vi "CC Data Logging Loop.vi"(11 "user event":refnum<user-event>) -> ()   [LabVIEW 2024]
uses:
  hk-channel-class/hk-channel-class/HK Table/HK Table.lvclass
  Subsystems/SS cluster Data Queue type.ctl
  CC enum Current Values Action.ctl
  Subsystems/SS cluster New Image Data.ctl
  typedefs/CC cluster Alarm Data.ctl
  typedefs/CC enum Alarm Action.ctl
  typedefs/CC cluster System Settings.ctl
  hk-channel-class/hk-channel-class/HK Item/HK Item.lvclass
panel:
  out "error out":errorcluster
  in  "error in (no error)":errorcluster
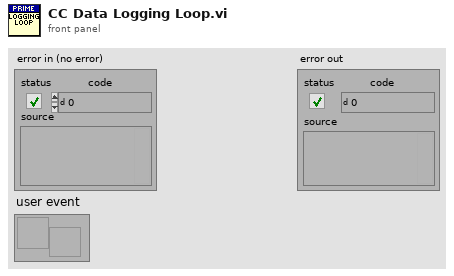
[diagram p1: front panel]
types:
  T1 = cluster{"HK Channels":refnum<class "HK Table.lvclass">, "Data Q":refnum<queue>, "user event":refnum<user-event>}
  T2 = typedef "CC enum Current Values Action.ctl" = enum16{"Init", "Write Item", "Write Array", "Read Item", "Read Array", "Read All", "Add Channels", "New File", "Add Message", "Get Current Values", "Close"}
  T3 = typedef "SS cluster New Image Data.ctl" = cluster{"Frame number":i32, "Detector #":u16, "FITS file":path, "File size":i64, "Image Type":string}
  T4 = typedef "CC enum Alarm Action.ctl" = enum16{"Init", "Add Alarm", "Get Alarms", "Clear Alarm", "Clear All Alarms"}
  T5 = typedef "CC cluster Alarm Data.ctl" = cluster{"Measured Value":dbl, "Alarm Low":dbl, "Alarm High":dbl, "Message":string, "Source":string}
  T6 = typedef "SS cluster Data Queue type.ctl" = cluster{"Source":string, "Type":string, "Data":variant}
  T7 = typedef "CC cluster System Settings.ctl" = cluster{"HK Table Name":string, "Images Folder":path, "Obs File":path}
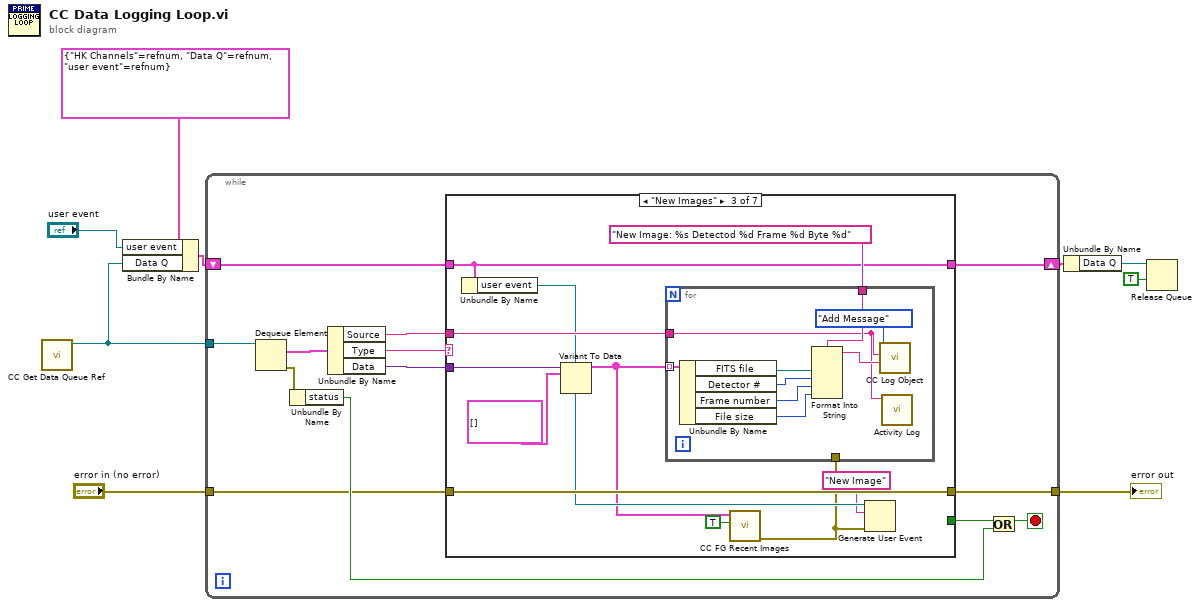
[diagram p0: block diagram]
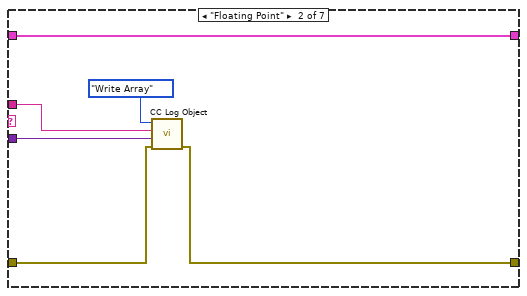
[diagram p3: hidden frame]
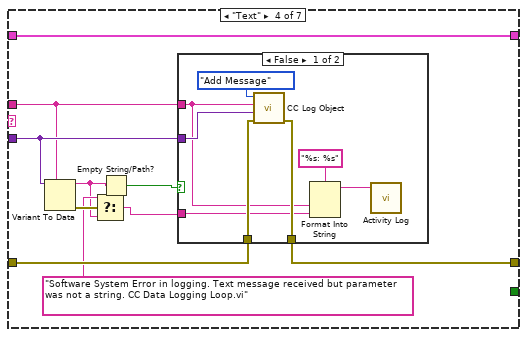
[diagram p4: hidden frame]
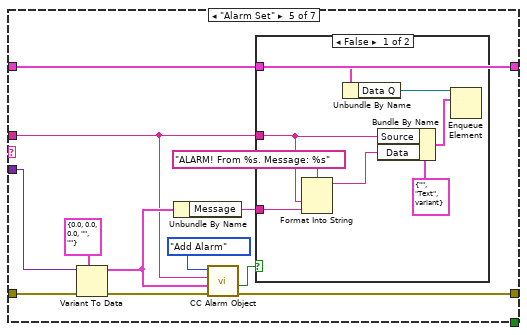
[diagram p6: hidden frame]
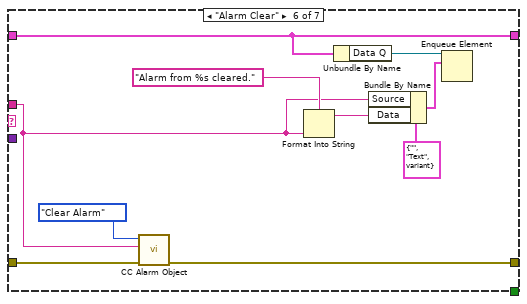
[diagram p8: hidden frame]
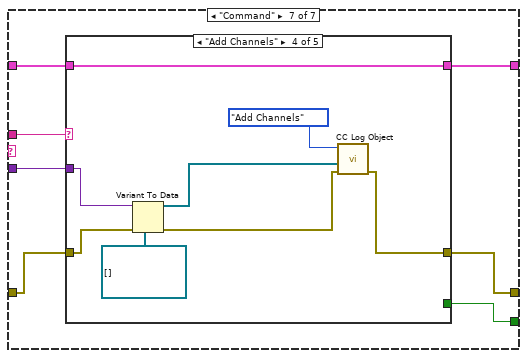
[diagram p9: hidden frame]
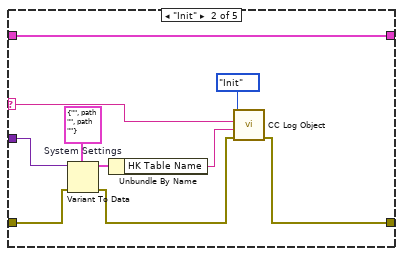
[diagram p11: hidden frame]
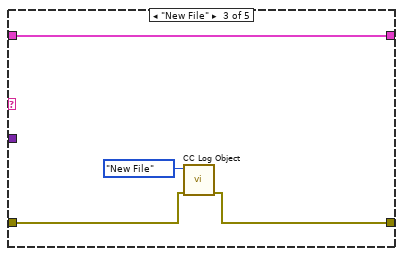
[diagram p12: hidden frame]
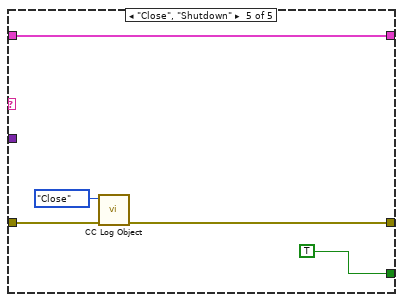
[diagram p13: hidden frame]
diagram:
  n1 = call "CC Get Data Queue Ref.vi"() -> ("Data Q"=w7:refnum<queue>)  [unwired: 10 in, 1 out]
  n2 = Bundle By Name(cluster=T1 {"HK Channels"=refnum, "Data Q"=refnum, "user event"=refnum}, "user event"="user event", "Data Q"=w7) -> (w5:T1)
  n3 = while {
    tunnel: w7 -> [w22]
    shift-right: [w12] -> w4
    shift-left: w5 -> [w16]
    tunnel: "error in (no error)" -> [w17]
    tunnel: [w11] -> w8
    stop <- w20 stop-if-true
    n4 = Dequeue Element(queue=w22) -> (element=w21:T6, error out=w19:errorcluster)  [unwired: 2 in, 2 out]
    n5 = Unbundle By Name(w19) -> ("status"=w18:bool)
    n6 = Unbundle By Name(w21) -> ("Source"=w14:string, "Type"=w15:string, "Data"=w13:variant)
    n7 = case shown="\"New Images\"" w15 {
      tunnel: w13 -> [_ w28 w41 w57 w80 _ w102]
      tunnel: w16 -> [w24 w27 w36 w60 w74 w90 w105]
      tunnel: [w24 w27 w36 w60 w74 w90 w104] -> w12
      tunnel: w14 -> [_ w29 w38 w56 w72 w89 w99]
      tunnel: w17 -> [w23 w26 w37 w59 w77 w96 w103]
      tunnel: [w23 w25 w37 w58 w75 w97 w101] -> w11
      tunnel: [_ _ _ _ _ _ w100] -> w10
      frame "False", Default {
      }
      frame "Floating Point" {
        n8 = call "CC Log Object.vi"("error in (no error)"=w26, "Data"=w28, "Source"=w29, "Action"=CC_enum_Current_Values_Action."Write Array") -> ("error out"=w25:errorcluster)  [unwired: 5 in, 2 out]
      }
      frame "New Images" {
        n9 = Unbundle By Name(w36) -> ("user event"=w35:refnum<user-event>)
        n10 = Variant To Data(type=T3[] [], Variant=w41) -> (data=w33:T3[])  [unwired: 1 in, 1 out]
        n11 = call "CC FG Recent Images.vi"("Write"=TRUE, "Recent Images"=w33) -> ("error out"=w31:errorcluster)  [unwired: 8 in, 1 out]
        n12 = for {
          tunnel: w33 -> [w50] mode=indexing
          tunnel: "New Image: %s Detectod %d Frame %d Byte %d" ("format string") -> [w49]
          tunnel: w38 -> [w42]
          tunnel: w31 -> [_]
          n13 = Unbundle By Name(w50) -> ("FITS file"=w48:path, "Detector #"=w47:u16, "Frame number"=w46:i32, "File size"=w45:i64)
          n14 = Format Into String(format string=w49, w48, w47, w46, w45) -> (resulting string=w43:string)  [unwired: 2 in, 1 out]
          n15 = call "CC Log Object.vi"("Data"=w43, "Source"=w42, "Action"=CC_enum_Current_Values_Action."Add Message") -> ()  [unwired: 6 in, 3 out]
          n16 = call "Activity Log.vi"("Message Log Entry"=w42) -> ()  [unwired: 9 in, 2 out]
        }
        n17 = Generate User Event(user event=w35, event data cluster="New Image" ("event data"), error in=w31) -> ()  [unwired: 1 in, 2 out]
      }
      frame "Text" {
        n18 = Variant To Data(type=w56, Variant=w57) -> (data=w52:string, error out=w55:errorcluster)  [unwired: 1 in]
        n19 = Select(t="Software System Error in logging. Text message received but parameter was not a string. CC Data Logging Loop.vi", s=w55, f=w52) -> (s? t:f=w54:string)
        n20 = Empty String/Path?(string/path=w52) -> (empty?=w51:bool)
        n21 = case shown="False" w51 {
          tunnel: w59 -> [w67 w69]
          tunnel: [w66 w69] -> w58
          tunnel: w57 -> [w65 _]
          tunnel: w56 -> [w63 _]
          tunnel: w54 -> [w61 _]
          frame False {
            n22 = call "CC Log Object.vi"("error in (no error)"=w67, "Data"=w65, "Source"=w63, "Action"=CC_enum_Current_Values_Action."Add Message") -> ("error out"=w66:errorcluster)  [unwired: 5 in, 2 out]
            n23 = Format Into String(format string="%s: %s", w63, w61) -> (resulting string=w62:string)  [unwired: 2 in, 1 out]
            n24 = call "Activity Log.vi"("Message Log Entry"=w62) -> ()  [unwired: 9 in, 2 out]
          }
          frame True {
          }
        }
      }
      frame "Alarm Set" {
        n25 = Variant To Data(error in=w77, type=T5 {"Measured Value"=0.0, "Alarm Low"=0.0, "Alarm High"=0.0, "Message"="", "Source"=""}, Variant=w80) -> (data=w73:T5, error out=w76:errorcluster)
        n26 = Unbundle By Name(w73) -> ("Message"=w71:string)
        n27 = call "CC Alarm Object.vi"("error in (no error)"=w76, "Alarm"=w73, "Source"=w72, "Alarm Action"=CC_enum_Alarm_Action."Add Alarm") -> ("error out"=w75:errorcluster, "key already included?"=w70:bool)  [unwired: 4 in, 2 out]
        n28 = case shown="False" w70 {
          tunnel: w74 -> [w88 _]
          tunnel: w72 -> [w83 _]
          tunnel: w71 -> [w82 _]
          frame False {
            n29 = Format Into String(format string="ALARM! From %s. Message: %s", w83, w82) -> (resulting string=w81:string)  [unwired: 2 in, 1 out]
            n30 = Unbundle By Name(w88) -> ("Data Q"=w87:refnum<queue>)
            n31 = Bundle By Name(cluster=T6 {"Source"="", "Type"="Text", "Data"=variant} ("element"), "Source"=w83, "Data"=w81) -> (w85:T6)
            n32 = Enqueue Element(queue=w87, element=w85) -> ()  [unwired: 2 in, 3 out]
          }
          frame True {
          }
        }
      }
      frame "Alarm Clear" {
        n33 = call "CC Alarm Object.vi"("error in (no error)"=w96, "Source"=w89, "Alarm Action"=CC_enum_Alarm_Action."Clear Alarm") -> ("error out"=w97:errorcluster)  [unwired: 5 in, 3 out]
        n34 = Format Into String(format string="Alarm from %s cleared.", w89) -> (resulting string=w91:string)  [unwired: 2 in, 1 out]
        n35 = Unbundle By Name(w90) -> ("Data Q"=w95:refnum<queue>)
        n36 = Bundle By Name(cluster=T6 {"Source"="", "Type"="Text", "Data"=variant} ("element"), "Source"=w89, "Data"=w91) -> (w93:T6)
        n37 = Enqueue Element(queue=w95, element=w93) -> ()  [unwired: 2 in, 3 out]
      }
      frame "Command" {
        n38 = case shown="\"Add Channels\"" w99 {
          selector: w99 -> [_ w114 _ _ _]
          tunnel: w105 -> [w106 w112 w121 w126 w134]
          tunnel: [w106 w112 w121 w126 w134] -> w104
          tunnel: w103 -> [w107 w108 w118 w124 w132]
          tunnel: [w107 w111 w119 w123 w131] -> w101
          tunnel: [_ _ _ _ TRUE] -> w100
          tunnel: w102 -> [_ w110 _ w122 _]
          frame "False", Default {
          }
          frame "Init" {
            w117 = T7 {"HK Table Name"="", "Images Folder"=path "", "Obs File"=path ""}  # System Settings
            n39 = Variant To Data(error in=w108, type=w117, Variant=w110) -> (data=w116:T7, error out=w109:errorcluster)
            n40 = Unbundle By Name(w116) -> ("HK Table Name"=w113:string)
            n41 = call "CC Log Object.vi"("error in (no error)"=w109, "Data"=w113, "Source"=w114, "Action"=CC_enum_Current_Values_Action."Init") -> ("error out"=w111:errorcluster)  [unwired: 5 in, 2 out]
          }
          frame "New File" {
            n42 = call "CC Log Object.vi"("error in (no error)"=w118, "Action"=CC_enum_Current_Values_Action."New File") -> ("error out"=w119:errorcluster)  [unwired: 7 in, 2 out]
          }
          frame "Add Channels" {
            n43 = Variant To Data(error in=w124, type=refnum<class "HK Item.lvclass">[] [], Variant=w122) -> (data=w127:refnum<class "HK Item.lvclass">[], error out=w125:errorcluster)
            n44 = call "CC Log Object.vi"("error in (no error)"=w125, "Data"=w127, "Action"=CC_enum_Current_Values_Action."Add Channels") -> ("error out"=w123:errorcluster)  [unwired: 6 in, 2 out]
          }
          frame "Close", "Shutdown" {
            n45 = call "CC Log Object.vi"("error in (no error)"=w132, "Action"=CC_enum_Current_Values_Action."Close") -> ("error out"=w131:errorcluster)  [unwired: 7 in, 2 out]
          }
        }
      }
    }
    n46 = Or(x=w10, y=w18) -> (x .or. y?=w20:bool)
  }
  "error out" <- w8
  n47 = Unbundle By Name(w4) -> ("Data Q"=w3:refnum<queue>)
  n48 = Release Queue(queue=w3, force destroy? (F)=TRUE) -> ()  [unwired: 1 in, 3 out]
